vi "PathPlanner_PathFinder_DoResetALT.vi"() -> (0 "Error":bool)   [LabVIEW 2019, in "PathPlanner24.lvlib"]
doc: "Internal function. Not to be used by end users."
uses:
  PathPlanner24.lvlib
  <vilib>/robotics/Navigation/shared/MapNode/OccupancyGridNode/NI_Robotics_OccupancyGridMapNode.lvclass
  C:/Program Files/National Instruments/LabVIEW 2019/vi.lib/robotics/Navigation/shared/MapNode/AbstractDstarNode/NI_Robotics_AbstractDstarNode.lvclass
  <vilib>/robotics/Navigation/shared/WorldMap/OccupancyGridWorldMap/NI_Robotics_OccupancyGridWorldMap.lvclass
  C:/Program Files/National Instruments/LabVIEW 2019/vi.lib/robotics/Navigation/shared/WorldMap/AbstractDstarWorldMap/NI_Robotics_AbstractDstarWorldMap.lvclass
  PathPlanner_PathFinder_Globals.vi
  <vilib>/robotics/Navigation/Anytime D Star/NI_Robotics_AnytimeDStar.lvclass
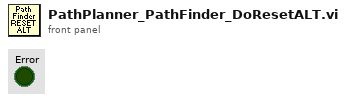
[diagram p1: front panel]
types:
  T1 = typedef "PathPlanner24.lvlib/PathPlannerFinderGridPosition.ctl" = cluster{"X":i32, "Y":i32}
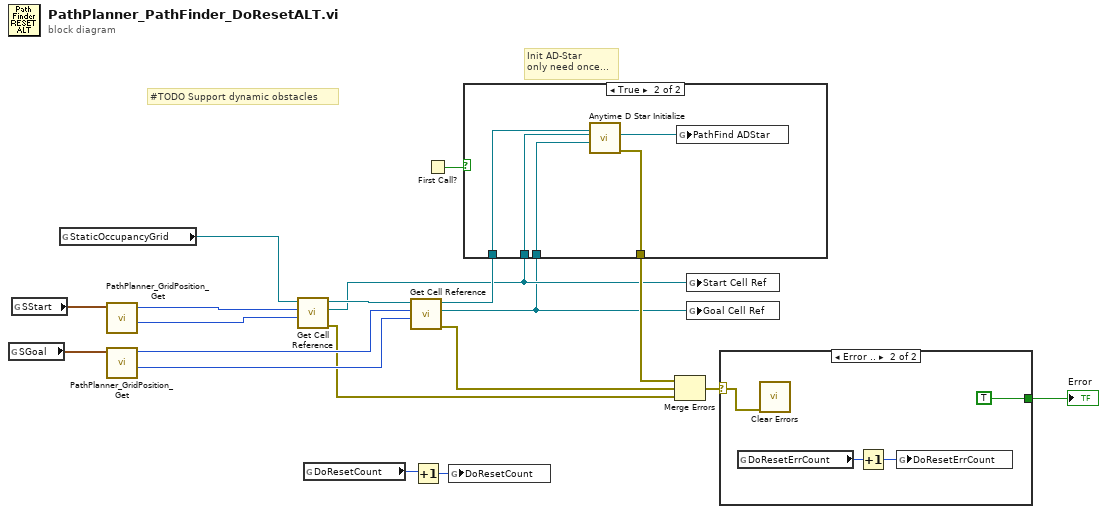
[diagram p0: block diagram]
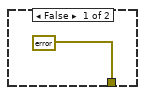
[diagram p2: hidden frame]
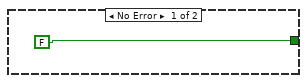
[diagram p3: hidden frame]
diagram:
  # "Init AD-Star\nonly need once..."
  # "#TODO Support dynamic obstacles"
  n1 = global read "PathPlanner_PathFinder_Globals.vi" "SGoal"() -> (w16:T1)
  n2 = global read "PathPlanner_PathFinder_Globals.vi" "SStart"() -> (w17:T1)
  n3 = global read "PathPlanner_PathFinder_Globals.vi" "StaticOccupancyGrid"() -> (w15:refnum<data-value>)
  n4 = call "PathPlanner_GridPosition_Get.vi"("GridPosition"=w17) -> ("Int Y"=w11:i32, "Int X"=w12:i32)  [unwired: 9 in]
  n5 = call "PathPlanner_GridPosition_Get.vi"("GridPosition"=w16) -> ("Int Y"=w9:i32, "Int X"=w10:i32)  [unwired: 9 in]
  n6 = call <vilib>:"Get Cell Reference.vi"("y"=w11, "x"=w12, "map reference in"=w15) -> ("error out"=w8:errorcluster, "cell reference"=w3:refnum<data-value>, "map reference out"=w14:refnum<data-value>)  [unwired: 5 in, 1 out]
  n7 = global read "PathPlanner_PathFinder_Globals.vi" "DoResetCount"() -> (w19:i64)
  n8 = call <vilib>:"Get Cell Reference.vi"("y"=w9, "x"=w10, "map reference in"=w14) -> ("error out"=w7:errorcluster, "cell reference"=w2:refnum<data-value>, "map reference out"=w13:refnum<data-value>)  [unwired: 5 in, 1 out]
  n9 = Increment(x=w19) -> (x+1=w18:i64)
  n10 = First Call?() -> (First Call?: T/F=w1:bool)
  n11 = global write "PathPlanner_PathFinder_Globals.vi" "DoResetCount"(w18) -> ()
  n12 = case shown="True" w1 {
    tunnel: w13 -> [_ w25]
    tunnel: [errorcluster {"status"=FALSE, "code"=0, "source"=""} ("error out") w23] -> w6
    tunnel: w3 -> [_ w22]
    tunnel: w2 -> [_ w21]
    frame False {
    }
    frame True {
      n13 = call <vilib>:"Anytime D Star Initialize.vi"("goal reference"=w21, "start reference"=w22, "map reference in"=w25) -> ("error out"=w23:errorcluster, "Anytime D*"=w24:refnum<class "NI_Robotics_AnytimeDStar.lvclass">)  [unwired: 7 in]
      n14 = global write "PathPlanner_PathFinder_Globals.vi" "PathFind ADStar"(w24) -> ()
    }
  }
  n15 = Merge Errors(w6, w7, w8) -> (w5:errorcluster)
  n16 = global write "PathPlanner_PathFinder_Globals.vi" "Start Cell Ref"(w3) -> ()
  n17 = global write "PathPlanner_PathFinder_Globals.vi" "Goal Cell Ref"(w2) -> ()
  n18 = case shown="Error .." w5 {
    selector: w5 -> [_ w27]
    tunnel: [FALSE TRUE] -> w4
    frame No Error {
    }
    frame Error {
      n19 = global read "PathPlanner_PathFinder_Globals.vi" "DoResetErrCount"() -> (w29:i64)
      n20 = call <vilib>:"Clear Errors.vi"("error in (no error)"=w27) -> ()  [unwired: 5 in, 2 out]
      n21 = Increment(x=w29) -> (x+1=w28:i64)
      n22 = global write "PathPlanner_PathFinder_Globals.vi" "DoResetErrCount"(w28) -> ()
    }
  }
  "Error" <- w4
